vi "Check.vi"() -> ()   [LabVIEW 2019]
uses:
  Z_Hswitch.xctl
  Y_source.ctl
  Heating.lvlib
panel:
  out "change":bool
  out "Boolean":bool
  in  "Z_Source":T1
  in  "connect":bool
  in  "Z_Hswitch":bool(xcontrol)
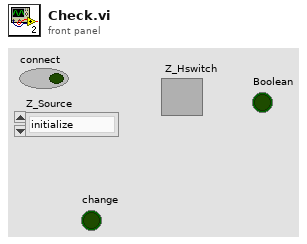
[diagram p1: front panel]
types:
  T1 = typedef "Heating.lvlib/Y_source.ctl" = enum8{"initialize", "local disabled", "local hand", "hand", "auto", "dist"}
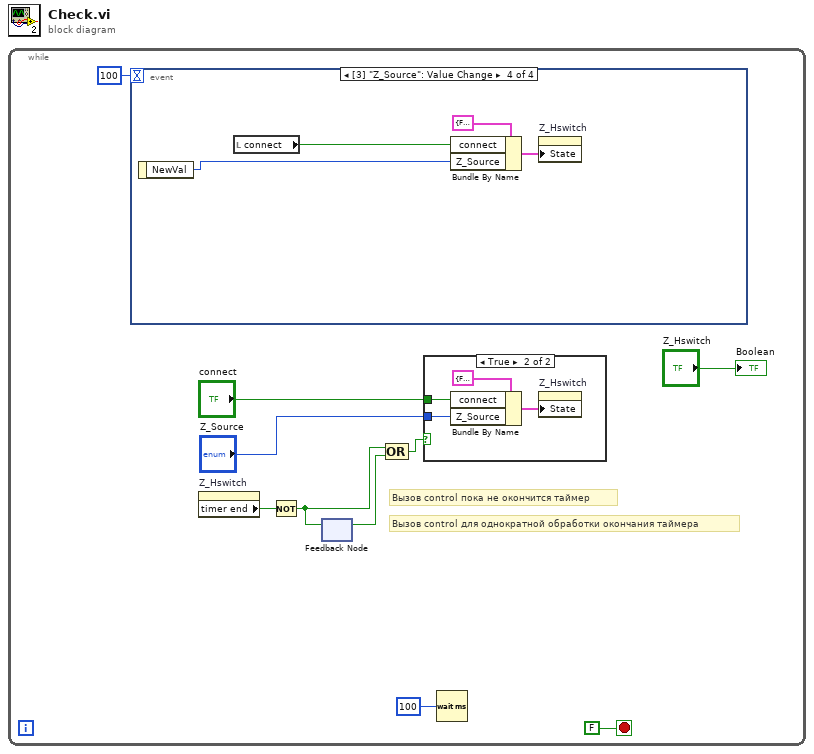
[diagram p0: block diagram]
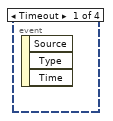
[diagram p2: hidden frame]
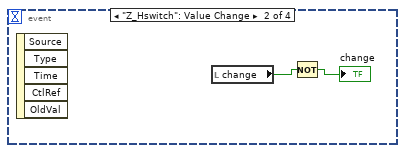
[diagram p3: hidden frame]
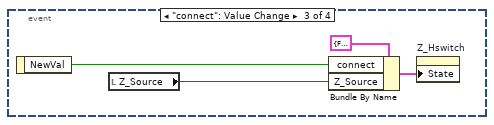
[diagram p4: hidden frame]
diagram:
  n1 = while {
    stop <- FALSE stop-if-true
    # "Вызов control пока не окончится таймер"
    # "Вызов control для однократной обработки окончания таймера"
    n2 = event shown="[3] \"Z_Source\": Value Change" {
      selector: _ -> [_ _ _ _]
      dyn-events: _ -> [_ _ _ _]
      timeout: 100 -> [_ _ _ _]
      event Timeout {
        n3 = event-data() -> ()  [unwired: 1 in, 3 out]
      }
      event "Z_Hswitch": Value Change {
        n4 = event-data() -> ()  [unwired: 1 in, 5 out]
        n5 = local read "change"() -> (w12:bool)
        n6 = Not(x=w12) -> (.not. x?=→"change":bool)
      }
      event "connect": Value Change {
        n7 = event-data() -> ("NewVal"=w16:bool)  [unwired: 1 in]
        n8 = local read "Z_Source"() -> (w13:T1)
        n9 = Bundle By Name(cluster=cluster{"connect":bool, "Z_Source":T1} {"connect"=FALSE, "Z_Source"=enum."initialize"} ("source"), "connect"=w16, "Z_Source"=w13) -> (w14:cluster{"connect":bool, "Z_Source":T1})
        n10 = property on="Z_Hswitch" class="Z_Hswitch (strict)"("State"=w14) -> ()  [unwired: 2 in, 2 out]
      }
      event Value Change {
        n11 = event-data() -> ("NewVal"=w17:T1)  [unwired: 1 in]
        n12 = local read "connect"() -> (w18:bool)
        n13 = Bundle By Name(cluster=cluster{"connect":bool, "Z_Source":T1} {"connect"=FALSE, "Z_Source"=enum."initialize"} ("source"), "connect"=w18, "Z_Source"=w17) -> (w19:cluster{"connect":bool, "Z_Source":T1})
        n14 = property on="Z_Hswitch" class="Z_Hswitch (strict)"("State"=w19) -> ()  [unwired: 2 in, 2 out]
      }
    }
    n15 = property on="Z_Hswitch" class="Z_Hswitch (strict)"() -> ("timer end"=w4:bool)  [unwired: 2 in, 2 out]
    n16 = Not(x=w4) -> (.not. x?=w2:bool)
    n17 = feedback-in #1(w2) -> ()
    n18 = feedback #1() -> (w3:bool)  [unwired: 1 in]
    n19 = Compound Arithmetic op=OR(w2, w3) -> (w8:bool)
    n20 = case shown="True" w8 {
      tunnel: "connect" -> [_ w23]
      tunnel: "Z_Source" -> [_ w22]
      frame False {
      }
      frame True {
        n21 = Bundle By Name(cluster=cluster{"connect":bool, "Z_Source":T1} {"connect"=FALSE, "Z_Source"=enum."initialize"} ("source"), "connect"=w23, "Z_Source"=w22) -> (w21:cluster{"connect":bool, "Z_Source":T1})
        n22 = property on="Z_Hswitch" class="Z_Hswitch (strict)"("State"=w21) -> ()  [unwired: 2 in, 2 out]
      }
    }
    n23 = Wait (ms)(milliseconds to wait=u32 100) -> ()  [unwired: 1 out]
    "Boolean" <- "Z_Hswitch"
  }
